vi "rszvl_quotedString_ReadCallback.vi"(5 "Attribute":T1={"Identifier"="", "Descriptive name"="", "Data Type"=enum."Integer 32", "Command"="", "Access"=2, "Range Table"="", "Read Callback"="", "Write Callback"="", "Range Callback"="", "Check Callback"="", "Rngtable Callback"="", "Coerce Callback"="", "Supported Models"="", "Instrument Options"="", "Repeated Capabilities"="", "Check Status Callback"="", "Index"=0, "Flag: OPC Wait"=FALSE, "Flag: Dont check status"=FALSE, "Flag: Cache Only"=FALSE} {"Access" items=["Read Only", "Write Only", "Read/Write"]}, 7 "Repeated Capability":string, 8 "error in":errorcluster, 11 "VISA resource name":refnum<visa-resource-name>) -> (0 "error out":errorcluster, 2 "Attribute Value String":string, 3 "VISA resource name out":refnum<visa-resource-name>)   [LabVIEW 2014]
uses:
  type_Attribute.ctl
  type_Attribute_Data_Type.ctl
  rszvl_rsidr_core.lvlib
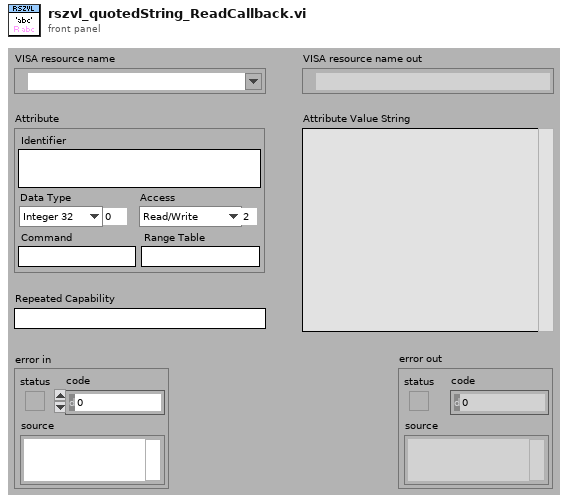
[diagram p1: front panel]
types:
  T1 = typedef "rszvl_rsidr_core.lvlib/type_Attribute.ctl" = cluster{"Identifier":string, "Descriptive name":string, "Data Type":T2, "Command":string, "Access":u16, "Range Table":string, "Read Callback":string, "Write Callback":string, "Range Callback":string, "Check Callback":string, "Rngtable Callback":string, "Coerce Callback":string, "Supported Models":string, "Instrument Options":string, "Repeated Capabilities":string, "Check Status Callback":string, "Index":i32, "Flag: OPC Wait":bool, "Flag: Dont check status":bool, "Flag: Cache Only":bool}
  T2 = typedef "rszvl_rsidr_core.lvlib/type_Attribute_Data_Type.ctl" = enum16{"Integer 32", "Double", "String", "Boolean", "None", "Integer 64"}
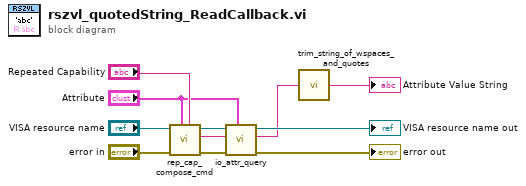
[diagram p0: block diagram]
diagram:
  n1 = call "rep_cap_compose_cmd.vi"("Repeated Capability"="Repeated Capability", "Attribute"="Attribute", "error in"="error in", "VISA resource name"="VISA resource name") -> ("error out"=w6:errorcluster, "Command out"=w8:string, "VISA resource name out"=w5:refnum<visa-resource-name>)  [unwired: 5 in]
  n2 = call "io_attr_query.vi"("Attribute"="Attribute", "error in"=w6, "write buffer"=w8, "VISA resource name"=w5) -> ("error out"=→"error out":errorcluster, "read buffer"=w1:string, "VISA resource name out"=→"VISA resource name out":refnum<visa-resource-name>)  [unwired: 5 in]
  n3 = call "trim_string_of_wspaces_and_quotes.vi"("String in"=w1) -> ("String out"=→"Attribute Value String":string)  [unwired: 4 in]
